vi "samplinginfo.vi"(5 "tone frequencies":dbl[](array[numeric]), 6 "Duration":dbl, 7 "Integer Degree of Nonlinearity":i64) -> (0 "sampling rate":dbl, 1 "Highest Frequency":dbl, 2 "Period of Lowest Frequency Input Tone":dbl, 3 "Lowest Frequency":dbl, 4 "# samples":dbl)   [LabVIEW 2009]
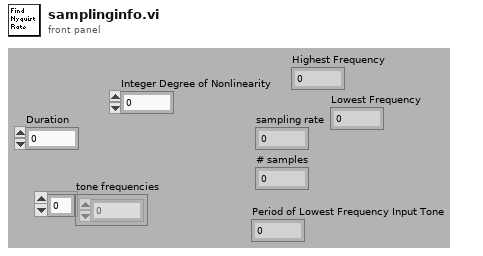
[diagram p1: front panel]
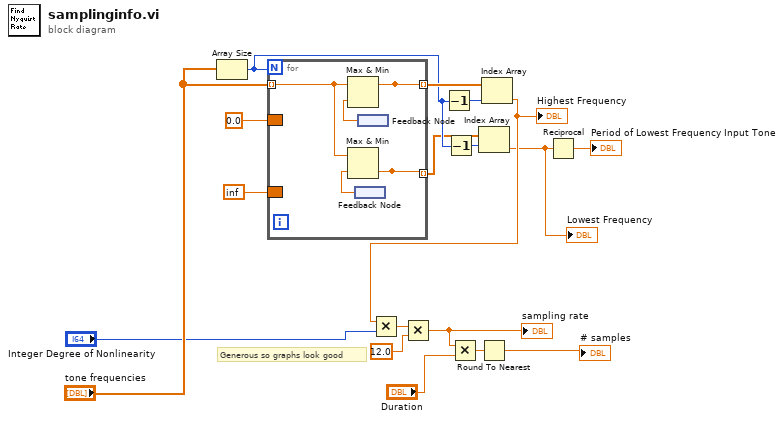
[diagram p0: block diagram]
diagram:
  # "Generous so graphs look good"
  n1 = Array Size(array="tone frequencies") -> (size(s)=w6:i32)
  n2 = for {
    N: w6 -> [_]
    tunnel: [w22] -> w17 mode=indexing
    tunnel: "tone frequencies" -> [w20] mode=indexing
    tunnel: [w19] -> w4 mode=indexing
    border: 0.0 -> [_]
    border: inf -> [_]
    n3 = feedback #1() -> (w21:dbl)
    n4 = Max & Min(x=w20, y=w21) -> (min(x,y)=w19:dbl)  [unwired: 1 out]
    n5 = feedback #2() -> (w23:dbl)
    n6 = Max & Min(x=w20, y=w23) -> (max(x,y)=w22:dbl)  [unwired: 1 out]
  }
  n7 = Decrement(x=w6) -> (x-1=w18:i32)
  n8 = Decrement(x=w6) -> (x-1=w7:i32)
  n9 = Index Array(array=w4, index=w7) -> (element=w3:dbl)
  "Lowest Frequency" <- w3
  n10 = Index Array(array=w17, index=w18) -> (element=w10:dbl)
  "Highest Frequency" <- w10
  n11 = Multiply(x=w10, y="Integer Degree of Nonlinearity") -> (x*y=w14:dbl)
  n12 = Multiply(x=w14, y=12.0) -> (x*y=w12:dbl)
  "sampling rate" <- w12
  n13 = Multiply(x=w12, y="Duration") -> (x*y=w13:dbl)
  n14 = Round To Nearest(number=w13) -> (nearest integer value=→"# samples":dbl)
  n15 = Reciprocal(x=w3) -> (1/x=→"Period of Lowest Frequency Input Tone":dbl)
